vi "Close Instrument.vi"(7 "Go Local (\"@LOC\")":bool, 8 "error in (no error)":errorcluster, 11 "Tektronix DPO MSO 2000 4000 in":refnum<class "Tektronix DPO MSO 2000 4000.lvclass">) -> (0 "error out":errorcluster, 3 "Tektronix DPO MSO 2000 4000 out":refnum<class "Tektronix DPO MSO 2000 4000.lvclass">)   [LabVIEW 2020, in "Tektronix DPO MSO 2000 4000.lvclass"]
uses:
  Tektronix DPO MSO 2000 4000.lvclass
  C:/Sandbox/RF Bench/Source Code/WiSpry Test Framework/Instruments/Instrument.lvclass
  Instrument.lvclass/Instrument.ctl
  Instrument.lvclass
  <instrlib>/Tektronix DPO MSO 2000 4000 Series/Tektronix DPO MSO 2000 4000 Series.lvlib
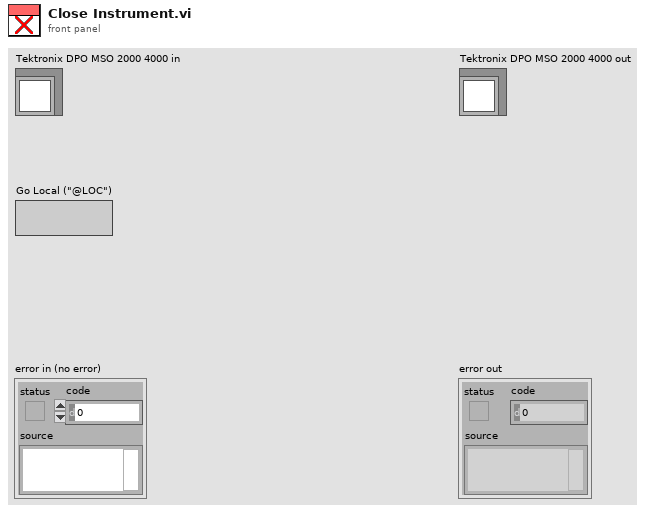
[diagram p1: front panel]
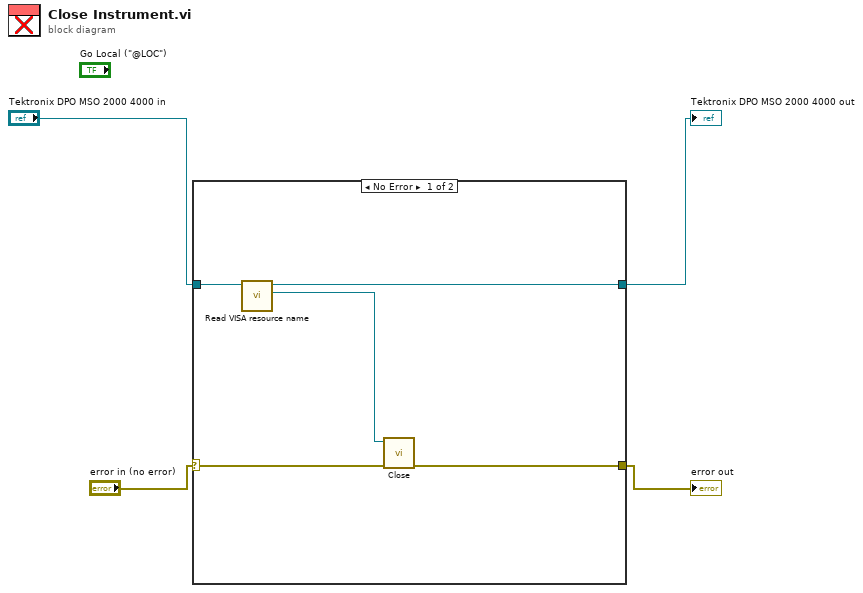
[diagram p0: block diagram]
diagram:
  n1 = case shown="No Error" "error in (no error)" {
    selector: "error in (no error)" -> [w7 w11]
    tunnel: [w6 w11] -> w2
    tunnel: [w8 w10] -> w1
    tunnel: "Tektronix DPO MSO 2000 4000 in" -> [w9 w10]
    frame No Error {
      n2 = call "Read VISA resource name.vi"("Instrument in"=w9) -> ("VISA resource name"=w5:refnum<visa-resource-name>, "Instrument out"=w8:refnum<class "Tektronix DPO MSO 2000 4000.lvclass">)  [unwired: 9 in]
      n3 = call <instrlib>:"Close.vi"("error in (no error)"=w7, "VISA resource name"=w5) -> ("error out"=w6:errorcluster)  [unwired: 9 in]
    }
    frame Error {
    }
  }
  "error out" <- w2
  "Tektronix DPO MSO 2000 4000 out" <- w1
